vi "Modular Optiscan Test.vi"() -> ()   [LabVIEW 2012]
panel:
  in  "Command":T1(ring)=enum."Move Absolute"
  in  "Parameter in":dbl[](array[numeric])
  out "Status out":bool[](array[boolean])
  out "Parameter out":dbl[](array[numeric])
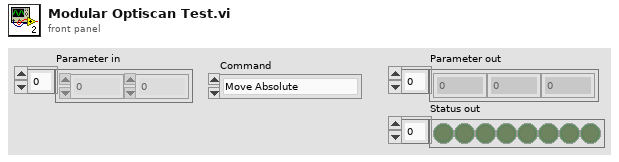
[diagram p1: front panel]
types:
  T1 = enum16{"Initialize", "Close", "Move Absolute", "Get Position", "Move Relative", "Set Acceleration", "Get Acceleration", "Set Speed", "Get Speed", "Limit Switch Status", "Motor Status", "Stop (controlled)", "Stop (instant)"}
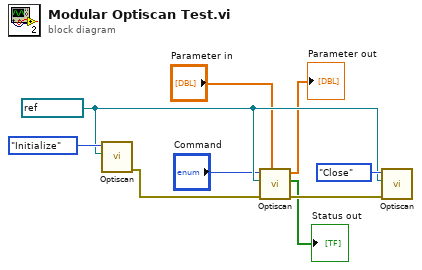
[diagram p0: block diagram]
diagram:
  w5 = refnum<visa-resource-name> "COM3" ("VISA resource name")
  n1 = call "Optiscan.vi"("VISA resource name"=w5, "Command"=T1."Initialize") -> ("error out"=w8:errorcluster)  [unwired: 4 in, 2 out]
  n2 = call "Optiscan.vi"("Parameter in"="Parameter in", "error in (no error)"=w8, "VISA resource name"=w5, "Command"="Command") -> ("error out"=w7:errorcluster, "Status out"=→"Status out":bool[], "Parameter out"=→"Parameter out":dbl[])  [unwired: 2 in]
  n3 = call "Optiscan.vi"("error in (no error)"=w7, "VISA resource name"=w5, "Command"=T1."Close") -> ()  [unwired: 3 in, 3 out]
